vi "Toggle Plugin.vi"(7 "menu reference":refnum<k9>, 8 "error in (no error)":errorcluster, 10 "Item Tag":string, 11 "Execution UI in":refnum<class "Execution UI.lvclass">) -> (0 "error out":errorcluster, 3 "Execution UI out":refnum<class "Execution UI.lvclass">)   [LabVIEW 2020, in "Execution UI.lvclass"]
uses:
  Execution UI.lvclass
  C:/git/astemes-lunit/source/User Interface/Process/Process.lvclass
  Process/Process.lvclass/Process.ctl
  Process/Process.lvclass
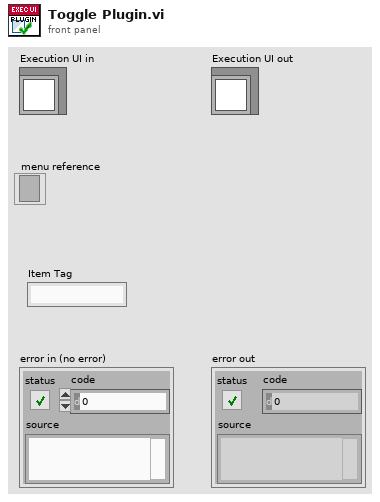
[diagram p1: front panel]
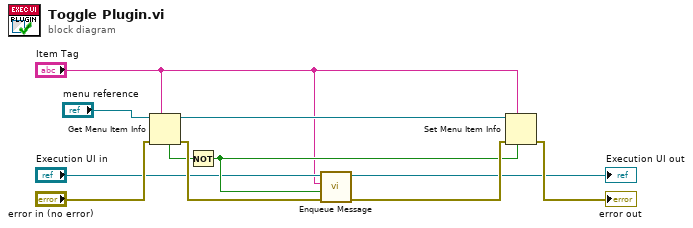
[diagram p0: block diagram]
diagram:
  n1 = Get Menu Item Info(7:"Item Tag", 8:"error in (no error)", 11:"menu reference") -> (0:w9:errorcluster, 3:w11:refnum<k9>, 4:w5:bool)  [unwired: 4 out]
  n2 = Not(x=w5) -> (.not. x?=w6:bool)
  n3 = call "Enqueue Message.vi"("error in (no error)"=w9, "Message Data"=w6, "Message"="Item Tag", "Process In"="Execution UI in") -> ("error out"=w7:errorcluster, "Process Out"=→"Execution UI out":refnum<class "Execution UI.lvclass">)  [unwired: 6 in]
  n4 = Set Menu Item Info(6:w6, 7:"Item Tag", 8:w7, 11:w11) -> (0:→"error out":errorcluster)  [unwired: 3 in, 1 out]
